vi "StringToU32array.vi"(3 "String":string) -> (0 "U32array":u32[](array[numeric]), 1 "size(Bytes)":i32, 2 "NumberElementsArrayU32":i32)   [LabVIEW 2015, in "VIPM2.lvlib"]
uses:
  VIPM2.lvlib
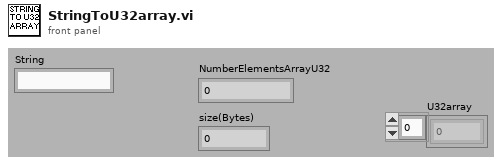
[diagram p1: front panel]
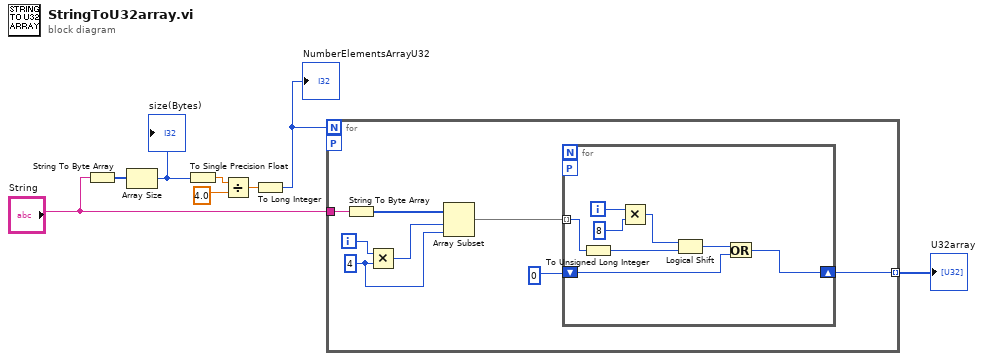
[diagram p0: block diagram]
diagram:
  n1 = String To Byte Array(string="String") -> (unsigned byte array=w5:u8[])
  n2 = Array Size(array=w5) -> (size(s)=w2:i32)
  "size(Bytes)" <- w2
  n3 = To Single Precision Float(number=w2) -> (single precision float=w3:sgl)
  n4 = Divide(x=w3, y=sgl 4.0) -> (x/y=w8:sgl)
  n5 = To Long Integer(number=w8) -> (32bit integer=w6:i32)
  "NumberElementsArrayU32" <- w6
  n6 = for {
    N: w6 -> [_]
    tunnel: [w9] -> w7 mode=indexing
    tunnel: "String" -> [w15]
    workers-P: _ -> [_]
    i -> [w11]
    w10 = 4 ("y")
    n7 = String To Byte Array(string=w15) -> (unsigned byte array=w14:u8[])
    n8 = Multiply(x=w11, y=w10) -> (x*y=w13:i32)
    n9 = Array Subset "Array Subset"(array=w14, index=w13, length=w10) -> (w12:u8[])
    n10 = for {
      shift-right: [w19] -> w9
      shift-left: u32 0 -> [w20]
      tunnel: w12 -> [w17] mode=indexing
      workers-P: _ -> [_]
      i -> [w24]
      n11 = To Unsigned Long Integer(number=w17) -> (unsigned 32bit integer=w18:u32)
      n12 = Multiply(x=w24, y=8) -> (x*y=w22:i32)
      n13 = Logical Shift(y=w22, x=w18) -> (x << y=w21:u32)
      n14 = Or(x=w21, y=w20) -> (x .or. y?=w19:u32)
    }
  }
  "U32array" <- w7
